vi "Cargo Control.vi"(10 "Operator Right Trigger":dbl, 11 "Operator Left Trigger":dbl) -> (2 "Numeric":dbl)   [LabVIEW 2018]
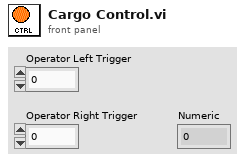
[diagram p1: front panel]
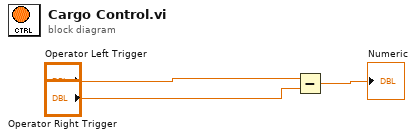
[diagram p0: block diagram]
diagram:
  n1 = Subtract(x="Operator Left Trigger", y="Operator Right Trigger") -> (x-y=→"Numeric":dbl)
